vi "ParserStringArrayToNumberArray(SubVI).vi"(1 "Array":string[](array[string])) -> (0 "Array 2":cluster{dbl[]}[][](array[cluster]))   [LabVIEW 2018]
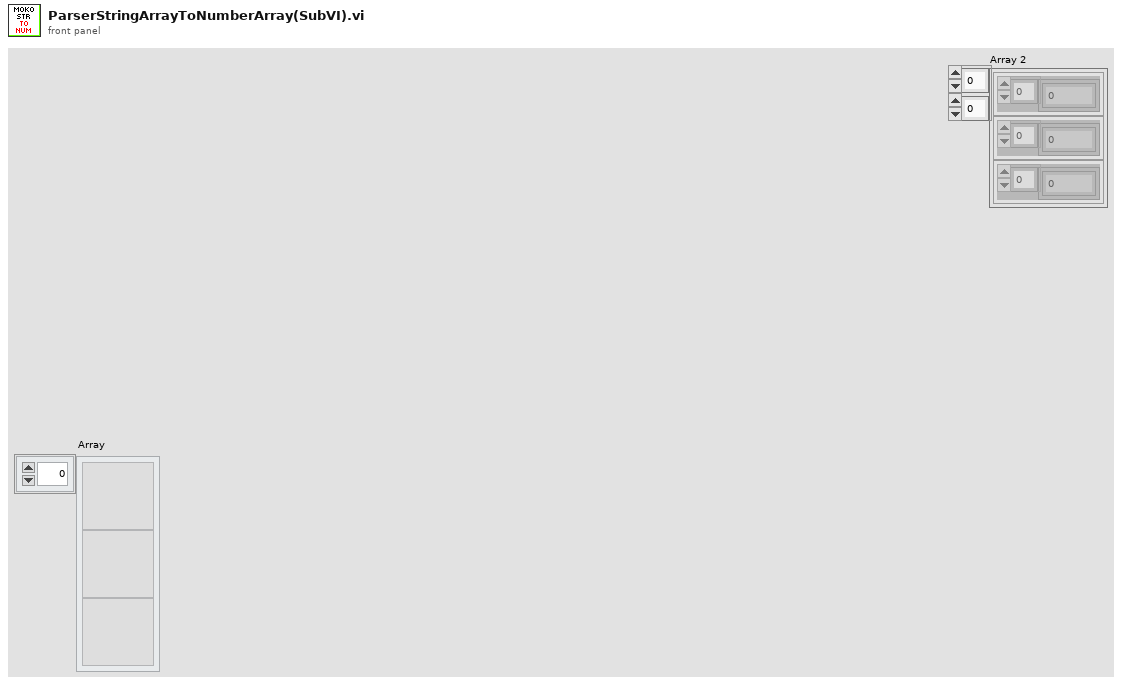
[diagram p1: front panel]
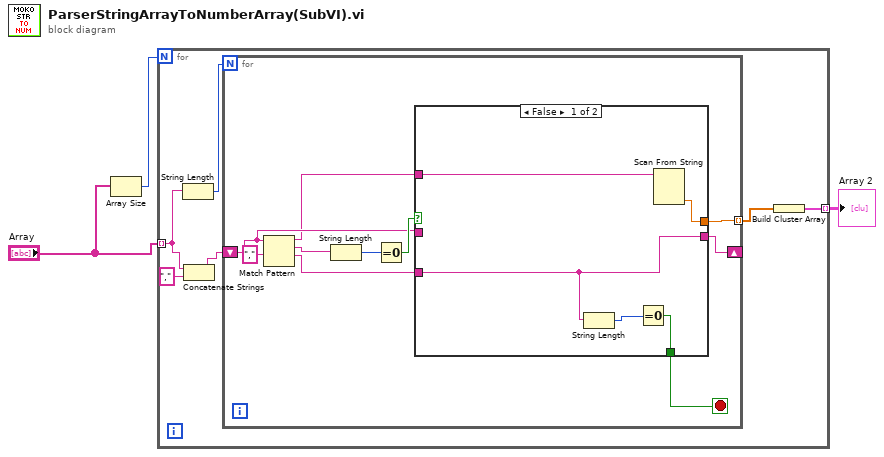
[diagram p0: block diagram]
diagram:
  n1 = Array Size(array="Array") -> (size(s)=w2:i32)
  n2 = for {
    N: w2 -> [_]
    tunnel: "Array" -> [w8] mode=indexing
    tunnel: [w4] -> w1 mode=indexing
    n3 = String Length(string=w8) -> (length=w9:i32)
    n4 = Concatenate Strings(w8, "," ("string")) -> (w6:string)
    n5 = for {
      N: w9 -> [_]
      shift-right: [w14] -> _
      shift-left: w6 -> [w15]
      tunnel: [w13] -> w5 mode=indexing
      stop <- w10 stop-if-true
      n6 = Match Pattern(string=w15, regular expression="," ("search string")) -> (before substring=w12:string, match substring=w18:string, after substring=w11:string)  [unwired: 1 in, 1 out]
      n7 = String Length(string=w18) -> (length=w17:i32)
      n8 = Equal To 0?(x=w17) -> (x = 0?=w16:bool)
      n9 = case shown="False" w16 {
        tunnel: w15 -> [_ w25]
        tunnel: [w22 w25] -> w14
        tunnel: [w24 _] -> w13
        tunnel: w12 -> [w23 _]
        tunnel: w11 -> [w22 _]
        tunnel: [w20 _] -> w10
        frame False {
          n10 = String Length(string=w22) -> (length=w21:i32)
          n11 = Equal To 0?(x=w21) -> (x = 0?=w20:bool)
          n12 = Scan From String(input string=w23) -> (output 1=w24:dbl)  [unwired: 4 in, 3 out]
        }
        frame True {
        }
      }
    }
    n13 = Build Cluster Array(w5) -> (w4:cluster{dbl[]}[])
  }
  "Array 2" <- w1
